vi "write config.vi"(8 "error in (no error)":errorcluster, 10 "value":cluster{"Boolean text":string, "Value":i32}[](array[cluster])) -> (0 "error out":errorcluster)   [LabVIEW 2020, in "Monedas.lvlib"]
doc: "write the configuration\n_____\nCreated using Delacor QMH Event Scripter 5.0.0.112."
uses:
  Monedas.lvlib
  <vilib>/Utility/xml.llb/Write to XML File(string).vi
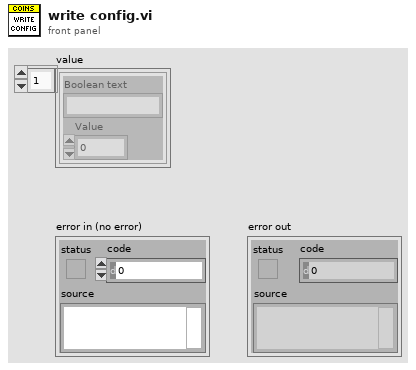
[diagram p1: front panel]
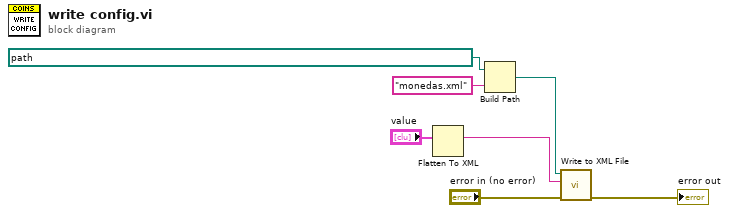
[diagram p0: block diagram]
diagram:
  n1 = Flatten To XML(6:"value") -> (2:w4:string)
  n2 = Build Path(base path=path "C:/Users/Ymata/Desktop/séptimo/labview 7mo/Proyecto máuina/Proyecto-maquina", name or relative path="monedas.xml") -> (appended path=w1:path)
  n3 = call-poly <vilib>:"Write to XML File.vi"("error in (no error)"="error in (no error)", "XML Input"=w4, "XML File Path"=w1) -> ("error out"=→"error out":errorcluster)  [unwired: 6 in, 2 out]
